vi "qSRA.vi"(0 "System no.":i32=1 min=1 max=4 step=1, 2 "Axes to query":string[](array[string]), 3 "All axes?":bool, 4 "Axis identifier?":bool=TRUE, 5 "error in":errorcluster) -> (14 "Gear ratio":dbl[](array[numeric]) format="%.6f", 19 "error out":errorcluster)   [LabVIEW 2020]
doc: "Returns gear ratio values for specified axes.\n\nC-843, C-848, C-880: If All axes = TRUE, then Axis identifier can be FALSE. This command can only be issued to a slave axis."
panel:
  # "Returns gear ratio values for specified axes."
  # "If all axes: use"
  # "Query"
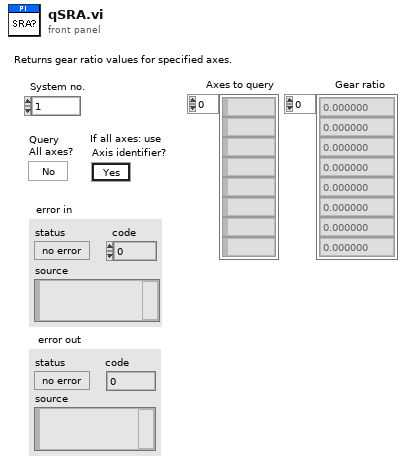
[diagram p1: front panel]
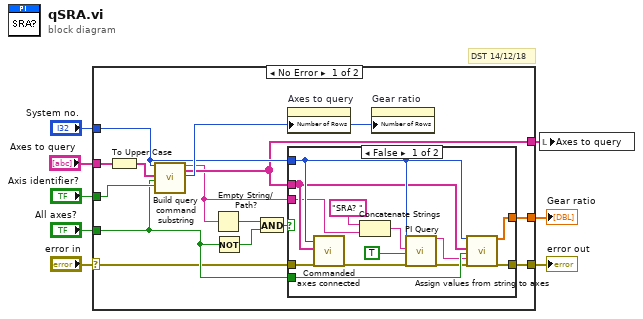
[diagram p0: block diagram]
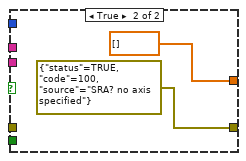
[diagram p2: hidden frame]
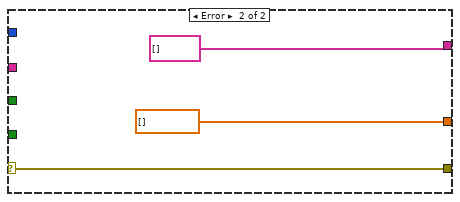
[diagram p3: hidden frame]
diagram:
  # "DST 14/12/18"
  n1 = case shown="No Error" "error in" {
    selector: "error in" -> [w9 w38]
    tunnel: [w22 dbl[] [] ("Values")] -> w8
    tunnel: "Axes to query" -> [w21 _]
    tunnel: [w20 w38] -> w6
    tunnel: "Axis identifier?" -> [w18 _]
    tunnel: "System no." -> [w16 _]
    tunnel: [w15 string[] [] ("Axes to query out")] -> w3
    tunnel: "All axes?" -> [w14 _]
    frame No Error {
      n2 = To Upper Case(1:w21) -> (0:w19:string[])
      n3 = call "Build query command substring.vi"("System no."=w16, "Axes to query in"=w19, "Query\nAll axes?"=w14, "For all axes: use\nAxis identifier?"=w18) -> ("Command substring"=w13:string, "Axes to query out"=w15:string[], "Number of rows"=w17:u32)  [unwired: 2 in, 11 out]
      n4 = Empty String/Path?(string/path=w13) -> (empty?=w12:bool)
      n5 = Not(x=w14) -> (.not. x?=w11:bool)
      n6 = And(x=w12, y=w11) -> (x .and. y?=w10:bool)
      n7 = property on="Axes to query" class="Arr (strict)"("Number of Rows"=w17) -> ()  [unwired: 2 in, 2 out]
      n8 = case shown="False" w10 {
        tunnel: [w32 dbl[] [] ("Values")] -> w22
        tunnel: w9 -> [w31 _]
        tunnel: [w27 errorcluster {"status"=TRUE, "code"=100, "source"="SRA? no axis specified"} ("error out")] -> w20
        tunnel: w16 -> [w30 _]
        tunnel: w15 -> [w29 _]
        tunnel: w14 -> [w28 _]
        tunnel: w13 -> [w25 _]
        frame False {
          n9 = call "Commanded axes connected.vi"("System no."=w30, "Commanded axes"=w29, "error in"=w31) -> ("error out"=w26:errorcluster)  [unwired: 1 in, 15 out]
          n10 = Concatenate Strings("SRA? ", w25) -> (w33:string)
          n11 = call "PI Query.vi"("System no."=w30, "String to send"=w33, "Attach termination char.?"=TRUE ("Attach Linefeed?"), "error in"=w26) -> ("String read"=w24:string, "error out"=w23:errorcluster)  [unwired: 3 in, 11 out]
          n12 = call "Assign values from string to axes.vi"("System no."=w30, "Queried axes"=w29, "All axes queried?"=w28, "Input String"=w24, "error in"=w23) -> ("Values"=w32:dbl[], "error out"=w27:errorcluster)  [unwired: 4 in, 9 out]
        }
        frame True {
        }
      }
      n13 = property on="Gear ratio" class="Arr (strict)"("Number of Rows"=w17) -> ()  [unwired: 2 in, 2 out]
    }
    frame Error {
    }
  }
  "error out" <- w6
  "Gear ratio" <- w8
  n14 = local write "Axes to query"(w3) -> ()
